vi "Get Environment.vi"(4 "출장교정 List":refnum<vi>, 6 "현장리스트?":bool, 7 "교정환경 in":T1, 8 "에러 입력(에러 없음)":errorcluster, 10 "교정정보 in":T2 caption="교정정보 입력 클러스터", 11 "참조 번호 입력":T3) -> (0 "에러 출력":errorcluster, 2 "교정정보 out":T2 caption="교정정보 출력 클러스터", 3 "참조 번호 출력":T3, 5 "교정환경out":T1 caption="교정환경 out")   [LabVIEW 2020]
uses:
  <vilib>/addons/database/Connection.llb/Conn ObjectReference.ctl
  Controls/Clst_Cal Info Global.ctl
  Controls/Clst_Atm Info Global.ctl
  Controls/Cmd_Read Query.ctl
  Controls/Clst_Query Info.ctl
  Public/Polymorph/ini Ctrl_1D Str.vi
  <vilib>/Utility/error.llb/Error Cluster From Error Code.vi
  <vilib>/ErrorRing/Error Ring.xnode
  <vilib>/addons/database/NI_Database_API.lvlib
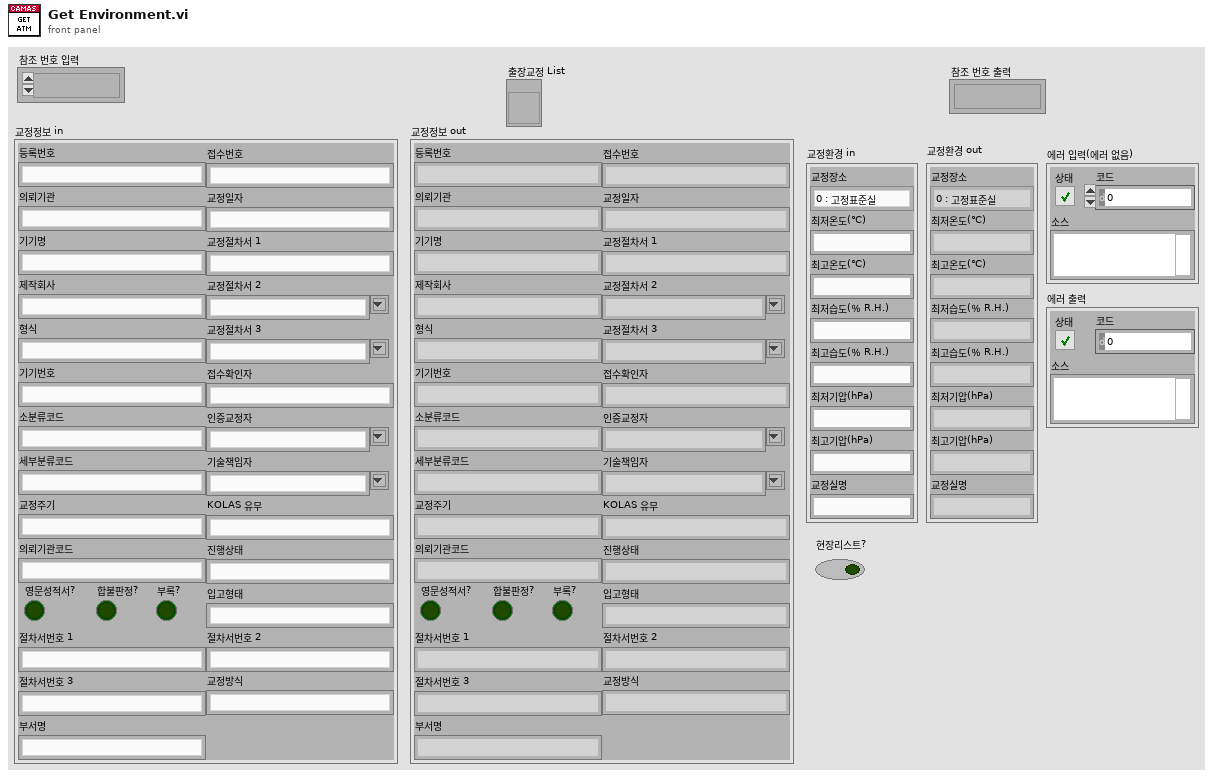
[diagram p1: front panel]
types:
  T1 = typedef "Clst_Atm Info Global.ctl" = cluster{"교정장소":enum16{"0 : 고정표준실", "1 : 현장교정"}, "최저온도(℃)":string, "최고온도(℃)":string, "최저습도(％ R.H.)":string, "최고습도(％ R.H.)":string, "최저기압(hPa)":string, "최고기압(hPa)":string, "교정실명":string}
  T2 = typedef "Clst_Cal Info Global.ctl" = cluster{"등록번호":string, "의뢰기관":string, "기기명":string, "제작회사":string, "형식":string, "기기번호":string, "소분류코드":string, "세부분류코드":string, "교정주기":string, "접수번호":string, "교정일자":string, "교정절차서 1":string, "교정절차서 2":string, "교정절차서 3":string, "접수확인자":string, "인증교정자":string, "기술책임자":string, "KOLAS 유무":string, "진행상태":string, "의뢰기관코드":string, "입고형태":string, "영문성적서?":bool, "합불판정?":bool, "부록?":bool, "절차서번호 1":string, "절차서번호 2":string, "절차서번호 3":string, "교정방식":string, "부서명":string}
  T3 = typedef "NI_Database_API.lvlib/Conn ObjectReference.ctl" = refnum<k1>
  T4 = typedef "Clst_Query Info.ctl" = cluster{"사번":string, "등록번호":string, "업체명":string, "세부분류코드":string, "형식":string, "기기번호":string, "FUNC":string, "FUNC_EXT":string, "옵션":string, "추가문자열":string, "일자":string, "배열 1":string[], "배열 2":string[], "항목명":string, "문자열":string, "이름":string}
  T5 = typedef "Cmd_Read Query.ctl" = enum16{"교정자 이름 얻기", "인증교정자 얻기", "기술책임자 얻기", "기책부책 얻기", "등록번호 얻기", "등록정보 얻기", "업체정보 얻기", "교정일자(CAMAS) 얻기", "교정일자(CALSTD) 얻기", "교정환경 얻기", "교정절차서 목록 얻기", "교정절차서명 얻기", "교정절차 목록얻기", "교정절차 얻기", "PROC 교정절차 얻기", "PROC SPEC 얻기", "교정절차(Func별) 얻기", "교정절차(Func_ext별) 얻기", "기관코드 얻기", "교정기능(세부분류) 얻기", "교정기능(모델) 얻기", "교정기능 목록 얻기", "교정기능 명칭 얻기", "교정기능 항목명칭 얻기", "DB (사용기준기) 얻기", "DB (기준기이름) 얻기", "DB (기준기이름목록) 얻기", "DB (기준기목록) 얻기", "DB (기준기값) 얻기", "DB (CMC) 얻기", "DB (FUNC) 얻기", "DB (CALNAME) 얻기", "DB (STDNAME) 얻기", "DB (SPEC) 얻기", "모델(항목전체) 얻기", "모델(최대범위) 얻기", "모델(최소범위) 얻기", "모델(최대최소) 얻기", "모델(범위조건) 얻기", "모델(등록요청) 얻기", "모델(형식별) 얻기", "모델(조건별) 얻기", "모델(모델검색) 얻기", "세부분류 목록 얻기", "기준기등록리스트 얻기", "STD Cal Date Check", "DB등록일자 얻기", "적용항목 얻기", "기타정보 얻기", "기준기요청 얻기", "서버버전 얻기"}
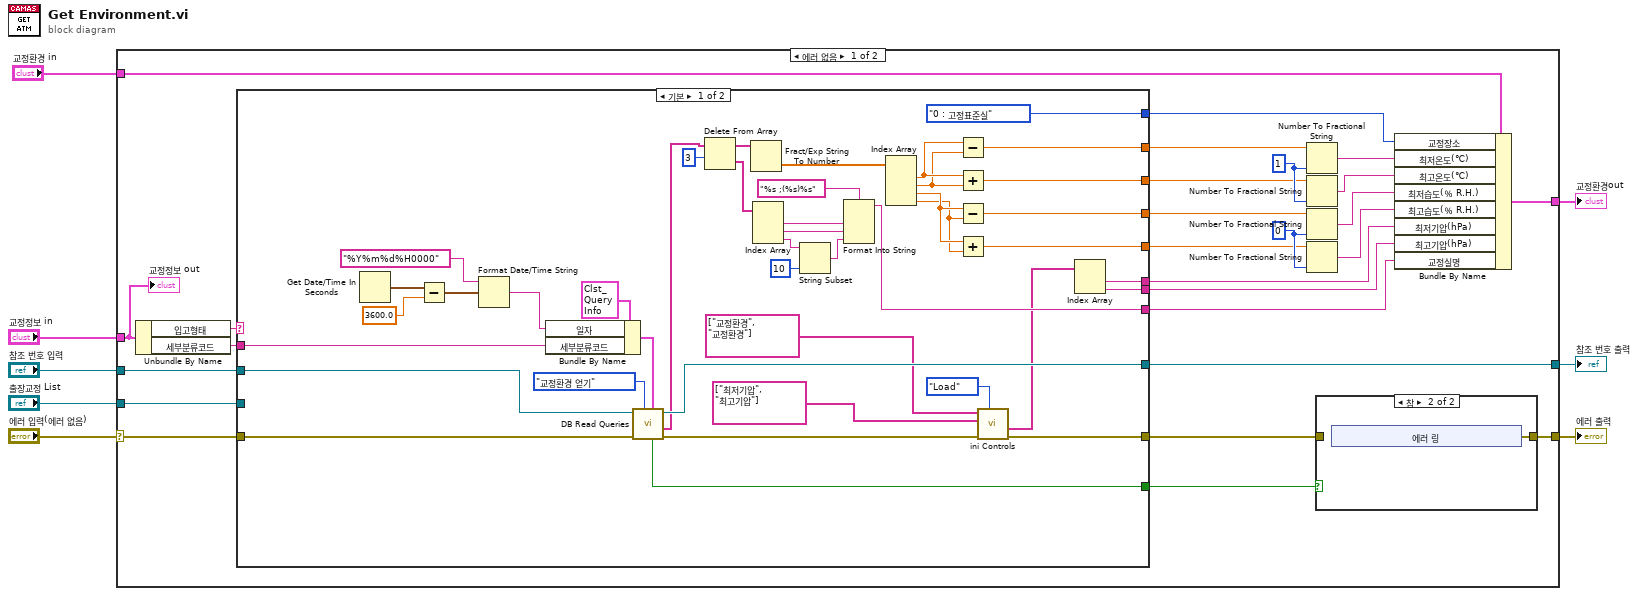
[diagram p0: block diagram]
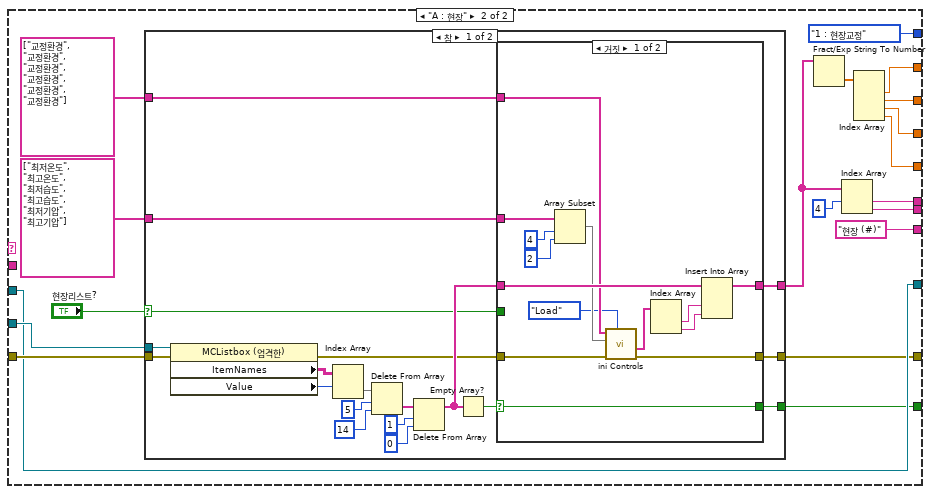
[diagram p3: hidden frame]
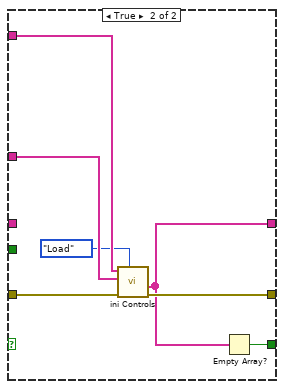
[diagram p4: hidden frame]
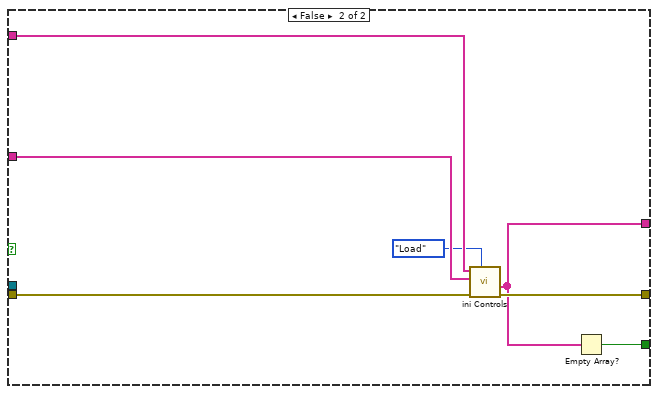
[diagram p5: hidden frame]
diagram:
  n1 = case shown="에러 없음" "에러 입력(에러 없음)" {
    selector: "에러 입력(에러 없음)" -> [w12 w152]
    tunnel: [w28 w150] -> w8
    tunnel: "교정정보 in" -> [w27 _]
    tunnel: "참조 번호 입력" -> [w24 w151]
    tunnel: [w18 w151] -> w5
    tunnel: "출장교정 List" -> [w17 _]
    tunnel: [w15 w152] -> w3
    tunnel: "교정환경 in" -> [w14 w150]
    frame No Error {
      w33 = i16 0 ("정밀도(6)")
      w34 = i16 1 ("정밀도(6)")
      n2 = Unbundle By Name(w27) -> ("입고형태"=w26:string, "세부분류코드"=w25:string)
      n3 = case shown="기본" w26 {
        tunnel: w25 -> [w42 _]
        tunnel: w12 -> [w83 w101]
        tunnel: w24 -> [w81 w94]
        tunnel: [w73 w98] -> w23
        tunnel: [w72 w97] -> w22
        tunnel: [w71 w96] -> w21
        tunnel: [w70 w95] -> w20
        tunnel: [enum16{"0 : 고정표준실", "1 : 현장교정"}."0 : 고정표준실" ("교정장소") enum16{"0 : 고정표준실", "1 : 현장교정"}."1 : 현장교정" ("교정장소")] -> w19
        tunnel: [w43 w91] -> w13
        tunnel: [w68 w94] -> w18
        tunnel: w17 -> [_ w100]
        tunnel: [w61 "현장 (#)" ("문자열")] -> w11
        tunnel: [w56 w92] -> w16
        tunnel: [w55 w87] -> w10
        tunnel: [w54 w86] -> w9
        frame Default {
          n4 = Get Date/Time In Seconds() -> (seconds since 1Jan1904=w53:timestamp)
          n5 = Subtract(x=w53, y=3600.0) -> (x-y=w51:timestamp)
          n6 = Format Date/Time String(time format string (%c)="%Y%m%d%H0000" ("시간 포맷 문자열 (%c)"), seconds (now)=w51) -> (date/time string=w49:string)  [unwired: 1 in]
          n7 = Bundle By Name(cluster=T4 {"사번"="", "등록번호"="", "업체명"="", "세부분류코드"="", "형식"="", "기기번호"="", "FUNC"="", "FUNC_EXT"="", "옵션"="", "추가문자열"="", "일자"="", "배열 1"=[], "배열 2"=[], "항목명"="", "문자열"="", "이름"=""} ("Query info"), "일자"=w49, "세부분류코드"=w42) -> (w79:T4)
          n8 = call "DB Read Queries.vi"("Query info"=w79, "Query Command"=Cmd_Read_Query."교정환경 얻기", "에러 입력(에러 없음)"=w83, "참조 번호 입력"=w81) -> ("에러 출력"=w45:errorcluster, "Data (0번행)"=w67:string[], "참조 번호 출력"=w68:T3, "None?"=w56:bool)  [unwired: 3 in, 1 out]
          n9 = Delete From Array(array=w67, length=3 ("길이")) -> (deleted portion=w64:string[], array with subset deleted=w66:string[])  [unwired: 1 in]
          n10 = Fract/Exp String To Number(string=w66) -> (number=w78:dbl[])  [unwired: 3 in, 1 out]
          n11 = Index Array(array=w64) -> (element #1=w63:string, element #2=w62:string, element #3=w59:string)  [unwired: 3 in]
          n12 = String Subset(string=w59, length (rest)=10 ("길이(나머지)")) -> (substring=w57:string)  [unwired: 1 in]
          n13 = Format Into String(format string="%s ;(%s)%s" ("포맷 문자열"), w63, w62, w57) -> (resulting string=w61:string)  [unwired: 2 in, 1 out]
          n14 = Index Array(array=w78) -> (element #1=w77:dbl, element #2=w76:dbl, element #3=w75:dbl, element #4=w74:dbl)  [unwired: 4 in]
          n15 = Subtract(x=w77, y=w76) -> (x-y=w73:dbl)
          n16 = Add(x=w77, y=w76) -> (x+y=w72:dbl)
          n17 = Subtract(x=w75, y=w74) -> (x-y=w71:dbl)
          n18 = Add(x=w75, y=w74) -> (x+y=w70:dbl)
          n19 = call-poly "ini Controls.vi"("Select"=enum16{"Save", "Load"}."Load", "에러 입력"=w45, "키"=string[] ["최저기압", "최고기압"], "섹션"=string[] ["교정환경", "교정환경"]) -> ("에러 출력"=w43:errorcluster, "값"=w44:string[])  [unwired: 5 in, 1 out]
          n20 = Index Array(array=w44) -> (element #1=w55:string, element #2=w54:string)  [unwired: 2 in]
        }
        frame "A : 현장" {
          n21 = case shown="참" "현장리스트?" {
            selector: "현장리스트?" -> [w103 _]
            tunnel: w101 -> [w113 w147]
            tunnel: w100 -> [w112 _]
            tunnel: [w109 w149] -> w92
            tunnel: [w108 w148] -> w91
            tunnel: string[] ["최저온도", "최고온도", "최저습도", "최고습도", "최저기압", "최고기압"] -> [w106 w146]
            tunnel: [w105 w145] -> w89
            tunnel: string[] ["교정환경", "교정환경", "교정환경", "교정환경", "교정환경", "교정환경"] -> [w104 w144]
            frame True {
              n22 = property class="MCListbox (엄격한)"(reference=w112, error in=w113) -> (error out=w107:errorcluster, "ItemNames"=w114:string[][], "Value"=w115:i32)  [unwired: 1 out]
              n23 = Index Array(array=w114, index (row)=w115) -> (element=w116:string[])  [unwired: 1 in]
              n24 = Delete From Array(array=w116, length=5 ("길이"), index=14 ("인덱스")) -> (deleted portion=w119:string[])  [unwired: 1 out]
              n25 = Delete From Array(array=w119, length=1 ("길이"), index=0 ("인덱스")) -> (array with subset deleted=w110:string[])  [unwired: 1 out]
              n26 = Empty Array?(array=w110) -> (empty?=w111:bool)
              n27 = case shown="거짓" w111 {
                selector: w111 -> [w135 _]
                tunnel: w107 -> [w127 w141]
                tunnel: [w123 w142] -> w108
                tunnel: w110 -> [w134 _]
                tunnel: [w133 w139] -> w105
                tunnel: w103 -> [_ _]
                tunnel: [w135 w140] -> w109
                tunnel: w106 -> [w132 w138]
                tunnel: w104 -> [w128 w137]
                frame False {
                  n28 = Array Subset(array=w132, index=4 ("인덱스"), length=2 ("길이")) -> (w129:string[])
                  n29 = call-poly "ini Controls.vi"("Select"=enum16{"Save", "Load"}."Load", "에러 입력"=w127, "키"=w129, "섹션"=w128) -> ("에러 출력"=w123:errorcluster, "값"=w126:string[])  [unwired: 5 in, 1 out]
                  n30 = Index Array(array=w126) -> (element #1=w125:string, element #2=w124:string)  [unwired: 2 in]
                  n31 = Insert Into Array(array=w134, new element #1=w125, new element #2=w124) -> (w133:string[])  [unwired: 1 in]
                }
                frame True {
                  n32 = call-poly "ini Controls.vi"("Select"=enum16{"Save", "Load"}."Load", "에러 입력"=w141, "키"=w138, "섹션"=w137) -> ("에러 출력"=w142:errorcluster, "값"=w139:string[])  [unwired: 5 in, 1 out]
                  n33 = Empty Array?(array=w139) -> (empty?=w140:bool)
                }
              }
            }
            frame False {
              n34 = call-poly "ini Controls.vi"("Select"=enum16{"Save", "Load"}."Load", "에러 입력"=w147, "키"=w146, "섹션"=w144) -> ("에러 출력"=w148:errorcluster, "값"=w145:string[])  [unwired: 5 in, 1 out]
              n35 = Empty Array?(array=w145) -> (empty?=w149:bool)
            }
          }
          n36 = Fract/Exp String To Number(string=w89) -> (number=w99:dbl[])  [unwired: 3 in, 1 out]
          n37 = Index Array(array=w89, index #1=4 ("인덱스")) -> (element #1=w87:string, element #2=w86:string)  [unwired: 1 in]
          n38 = Index Array(array=w99) -> (element #1=w98:dbl, element #2=w97:dbl, element #3=w96:dbl, element #4=w95:dbl)  [unwired: 4 in]
        }
      }
      n39 = Number To Fractional String(number=w23, precision (6)=w34) -> (F-format string=w32:string)  [unwired: 2 in]
      n40 = Number To Fractional String(number=w22, precision (6)=w34) -> (F-format string=w31:string)  [unwired: 2 in]
      n41 = Number To Fractional String(number=w21, precision (6)=w33) -> (F-format string=w30:string)  [unwired: 2 in]
      n42 = Number To Fractional String(number=w20, precision (6)=w33) -> (F-format string=w29:string)  [unwired: 2 in]
      n43 = case shown="참" w16 {
        tunnel: w13 -> [w35 _]
        tunnel: [w35 w36] -> w15
        frame False {
        }
        frame True {
          n44 = xnode "에러 링"() -> ("에러 출력"=w36:errorcluster)
        }
      }
      n45 = Bundle By Name(cluster=w14, "교정장소"=w19, "최저온도(℃)"=w32, "최고온도(℃)"=w31, "최저습도(％ R.H.)"=w30, "최고습도(％ R.H.)"=w29, "최저기압(hPa)"=w10, "최고기압(hPa)"=w9, "교정실명"=w11) -> (w28:T1)
      "교정정보 out" <- w27
    }
    frame Error {
    }
  }
  "에러 출력" <- w3
  "참조 번호 출력" <- w5
  "교정환경out" <- w8
